vi "start.vi"(8 "error in (no error)":errorcluster, 10 "Parameters":T1, 11 "Context in":refnum<class "Context.lvclass">) -> (0 "error out":errorcluster, 3 "Context out":refnum<class "Context.lvclass">)   [LabVIEW 2016, in "Context.lvclass"]
uses:
  Context.lvclass
  Communicator/Topics/CommandStart.ctl
  Communicator/Topics/CommandId.ctl
  Context.lvclass/Context.ctl
  States/State/State.lvclass
  Model/Model.lvclass
  Communicator/M1M3Communicator.lvlib
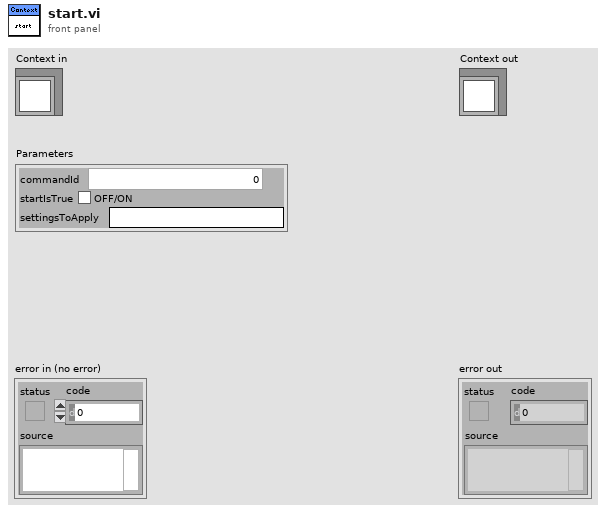
[diagram p1: front panel]
types:
  T1 = typedef "M1M3Communicator.lvlib/CommandStart.ctl" = cluster{"commandId":T2, "startIsTrue":bool, "settingsToApply":string}
  T2 = typedef "M1M3Communicator.lvlib/CommandId.ctl" = i32
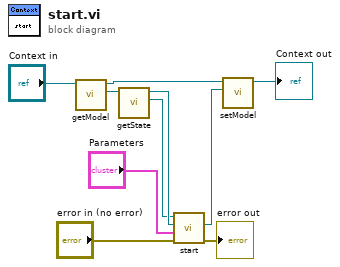
[diagram p0: block diagram]
diagram:
  n1 = call "getModel.vi"("Context in"="Context in") -> ("Model"=w3:refnum<class "Model.lvclass">, "Context out"=w5:refnum<class "Context.lvclass">)  [unwired: 9 in]
  n2 = call "getState.vi"("Model in"=w3) -> ("State out"=w9:refnum<class "State.lvclass">, "Model out"=w10:refnum<class "Model.lvclass">)  [unwired: 8 in, 1 out]
  n3 = call-dynamic "start.vi"("error in (no error)"="error in (no error)", "Parameters"="Parameters", "Model in"=w10, "State in"=w9) -> ("error out"=→"error out":errorcluster, "Model out"=w2:refnum<class "Model.lvclass">)  [unwired: 5 in, 1 out]
  n4 = call "setModel.vi"("Model"=w2, "Context in"=w5) -> ("Context out"=→"Context out":refnum<class "Context.lvclass">)  [unwired: 9 in]
